vi "joystick and camera_ms.vi"(9 "Tab Control":T2(tab)=enum."motion 2", 10 "Text":string, 11 "controller in":T5={"A3200.lvclass"=refnum, "Ultimus V2.lvclass"=refnum, "NI-DAQ.lvclass"=refnum, "Motion.lvclass"=refnum, "I-O.lvclass"=refnum, "Dispenser.lvclass"=refnum}) -> (2 "Gantry":dbl[](array[numeric]) format="%#_8g", 3 "controller out":T5)   [LabVIEW 2016]
uses:
  Classes/Controller/Motion/A3200 Folder/A3200.lvclass
  D:/Gantry_General/Classes/Controller/Motion/Motion Folder/Motion.lvclass
  Classes/Controller/Dispenser/Ultimus V2 Folder/Ultimus V2.lvclass
  Classes/Controller/I-O/NI-DAQ Folder/NI-DAQ.lvclass
  Classes/Controller/Motion/Motion Folder/Motion.lvclass
  Classes/Controller/I-O/I-O Folder/I-O.lvclass
  Classes/Controller/Dispenser/Dispenser Folder/Dispenser.lvclass
  Classes/Controller/Camera/Camera Folder/Machine Vision.ctl
  Classes/Controller/Camera/Camera Folder/Camera.lvclass
panel:
  out "pass/>(r)/<(-r)":bool[][](array[boolean])
  in  "range(r)":dbl[](array[numeric])=[0.001, 0.001, 0.0, 0.0] format="%#_8g"
  in  "camera on":bool
  in  "Go Gantry position":bool
  out "Gantry poistion":dbl[](array[numeric]) format="%#_8g"
  out "Boolean":bool
  in  "Machine Vision 2":T1=enum."tracker fiducial"
  in  "Machine Vision":T1=enum."None"
  in  "Joystick":bool
  in  "Go sum":bool
  out "Sum":dbl[](array[numeric])=[0.00017791618301998824, 0.0005389674915932119, 0.0, 0.0] format="%#_8g"
  out "Camera":dbl[](array[numeric])=[0.00017791618301998824, 0.0005389674915932119] format="%#_8g"
  in  "Stop":bool
  out "Numeric":dbl
  in  "input":dbl=70.0
  in  "Camera light":bool
  in  "On/Off":bool
  in  "Channel":i32=20
  in  "Vacuum":bool
  in  "Jog Cluster":T3={"Jog XY Cluster"={"object goes up"=FALSE, "object goes down"=FALSE, "object goes right"=FALSE, "object goes left"=FALSE, "SW2"=TRUE, "SW1"=TRUE, "YY (mm)"=0.1, "YN (mm) "=0.01, "NY (mm) "=0.002, "NN (mm) "=0.0005}, "Jog Z Cluster "={"Z go down 0.1 mm"=FALSE, "Z go up 0.1 mm"=FALSE, "Z go down 0.05 mm"=FALSE, "Z go up 0.05 mm"=FALSE, "Z go down 0.01 mm"=FALSE, "Z go up 0.01 mm"=FALSE, "Z go down"=FALSE, "Z go up"=FALSE, "step (mm)"=0.001}}
  in  "XY Speed 2":dbl=20.0
  in  "XY add":dbl[](array[numeric])=[380.0238, 0.0014, 55.58184794305402, -0.0005137759006832702] format="%#_8g"
  in  "get P2 add":bool
  in  "XY go 5":bool
  in  "XY Position 5":dbl[](array[numeric])=[389.0, 389.0, 55.58184800408918, -0.0005138406154977592] format="%#_8g"
  in  "get Postion 5":bool
  in  "XY go 4":bool
  in  "XY Position 4":dbl[](array[numeric])=[592.3687645323295, 397.60426466601484, 55.58184800408918, -0.0005138406154977592] format="%#_8g"
  in  "get Postion 4":bool
  in  "XY go 3":bool
  in  "XY Position 3":dbl[](array[numeric])=[972.3689967686571, 397.60610398471965, 55.58184796594221, -0.0005142432854545792] format="%#_8g"
  in  "get Postion 3":bool
  in  "XY Position 1":dbl[](array[numeric])=[9.0, 9.0, 35.37118150994465, -9.480284627999261e-05] format="%#_8g"
  in  "XY go 1":bool
  in  "Z Position":dbl=35.37
  in  "Z Go":bool
  in  "XY go 2":bool
  in  "XY Position 2":dbl[](array[numeric])=[769.0237955548766, 389.000010557689, 90.95302945299866, -0.0006085787469632629] format="%#_8g"
  in  "get Postion 1":bool
  in  "get Postion 2":bool
  in  "XY Speed":dbl=100.0
  in  "z Speed":dbl=20.0 format="%#_13g"
  in  "add postion":dbl[](array[numeric])=[360.0223, 0.0021, 0.0, 0.0] format="%#_8g"
  in  "get and go Position":T4={"get P Array"=[FALSE, FALSE, FALSE, FALSE, FALSE], "XY go P Array"=[FALSE, FALSE, FALSE, FALSE, FALSE], "xyzu Position Array"=[[369.99999758410644, 730.0222975841064, 0.0, 0.0, 370.0], [370.00000242422084, 370.0021024242208, 0.0, 0.0, 370.0], [35.29999980758057, 35.29999980758057, 0.0, 0.0, 35.3], [-6.534758156392827e-07, -6.534758156392827e-07, 0.0, 0.0, 0.0]], "XYZ go P Array"=[FALSE, FALSE, FALSE, FALSE, FALSE]} {"xyzu Position Array" format="%#_8g"}
  in  "input postion test":dbl[](array[numeric])
  out "Array out":dbl[](array[numeric])=[369.99999758410644, 370.00000242422084]
  out "XY(F)/XYZ(T)":bool
  in  "P2 get P1 add position":bool
  out "Image 2":T6(plugin-control)
  out "Image":T6(plugin-control)
  # "X\nY"
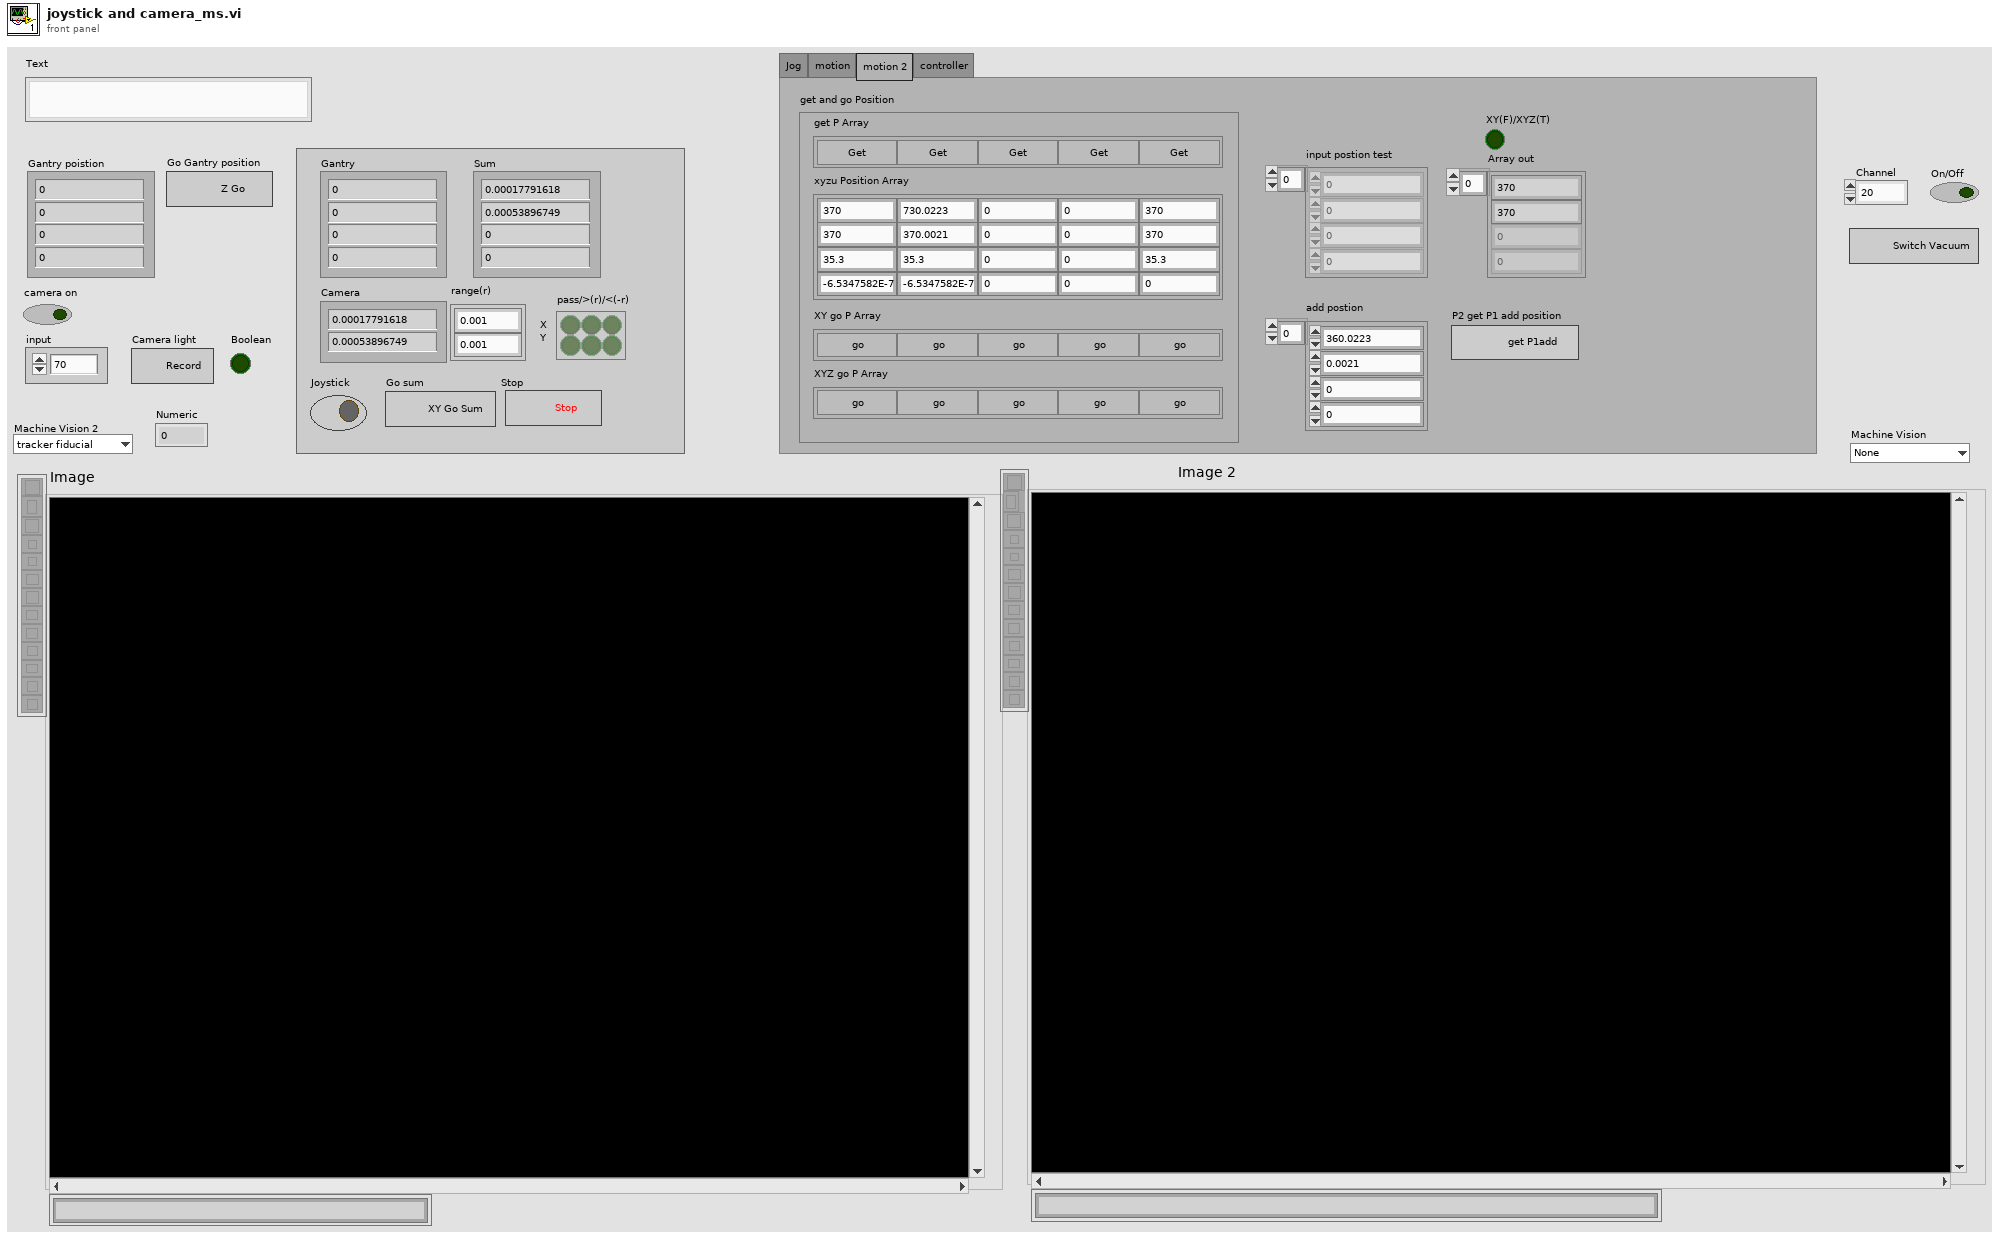
[diagram p1: front panel]
types:
  T1 = typedef "Camera.lvclass/Machine Vision.ctl" = enum16{"top left corner", "top right corner", "bottom left corner", "bottom right corner", "bottom left chip", "top right chip", "None", "tracker fiducial", "chip cross 2", "chip cross", "Focus", "INTT HDI Mark", "INTT Sensor Cross", "INTT Chip Corner", "HPK Silicon", "HPK Silicon square", "8inch PCB Pad ", "8inch PCB Pad2", "Circle", "tpcb_hole"}
  T2 = enum32{"Jog", "motion", "motion 2", "controller"}
  T3 = cluster{"Jog XY Cluster":cluster{"object goes up":bool, "object goes down":bool, "object goes right":bool, "object goes left":bool, "SW2":bool, "SW1":bool, "YY (mm)":dbl, "YN (mm) ":dbl, "NY (mm) ":dbl, "NN (mm) ":dbl}, "Jog Z Cluster ":cluster{"Z go down 0.1 mm":bool, "Z go up 0.1 mm":bool, "Z go down 0.05 mm":bool, "Z go up 0.05 mm":bool, "Z go down 0.01 mm":bool, "Z go up 0.01 mm":bool, "Z go down":bool, "Z go up":bool, "step (mm)":dbl}}
  T4 = cluster{"get P Array":bool[], "XY go P Array":bool[], "xyzu Position Array":dbl[][], "XYZ go P Array":bool[]}
  T5 = cluster{"A3200.lvclass":refnum<class "A3200.lvclass">, "Ultimus V2.lvclass":refnum<class "Ultimus V2.lvclass">, "NI-DAQ.lvclass":refnum<class "NI-DAQ.lvclass">, "Motion.lvclass":refnum<class "Motion.lvclass">, "I-O.lvclass":refnum<class "I-O.lvclass">, "Dispenser.lvclass":refnum<class "Dispenser.lvclass">}
  T6 = typedef "IMAQ Image.ctl" = refnum<image>
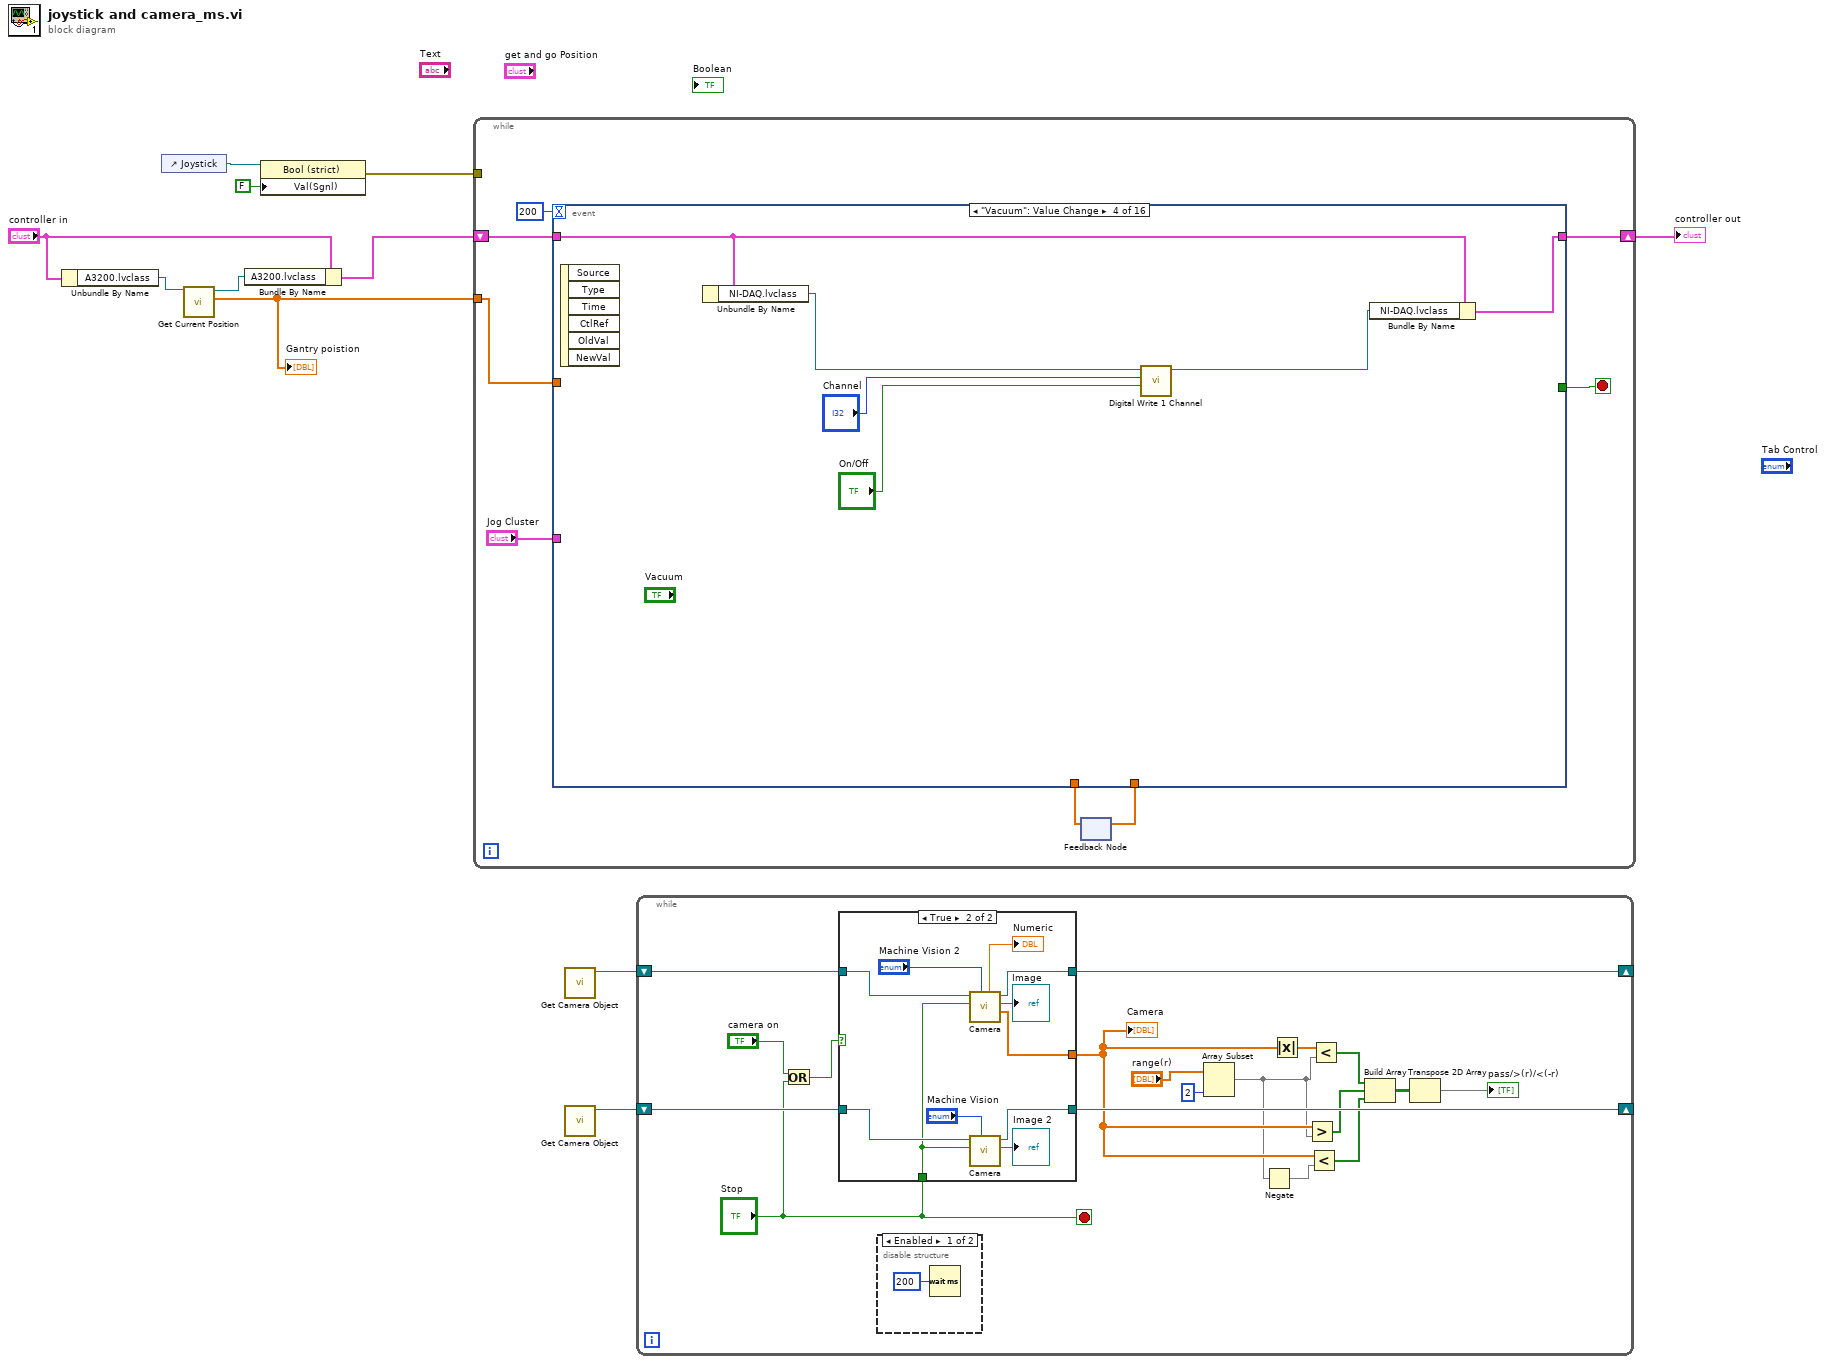
[diagram p0: block diagram]
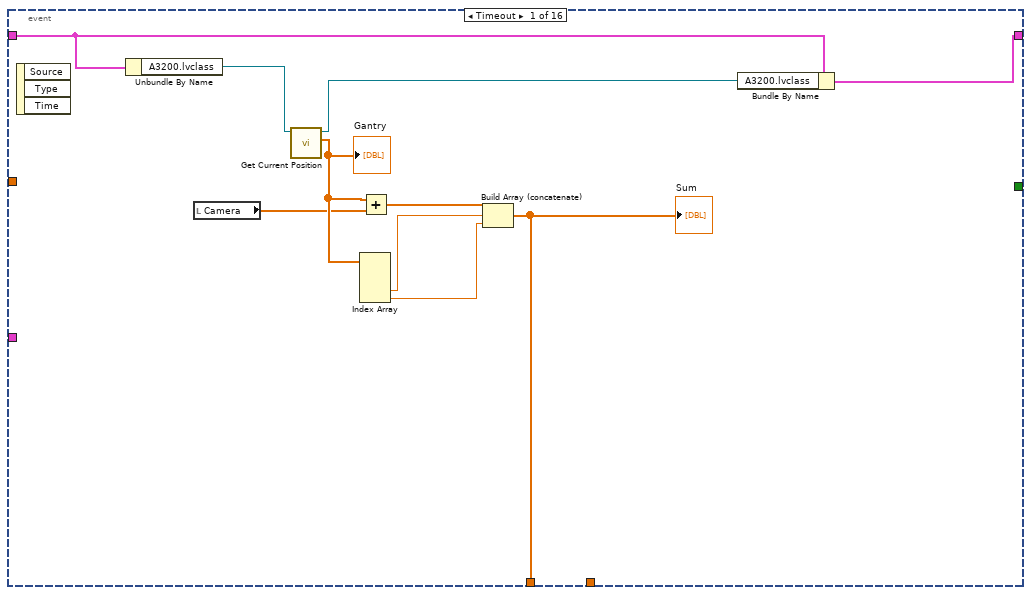
[diagram p2: hidden frame]
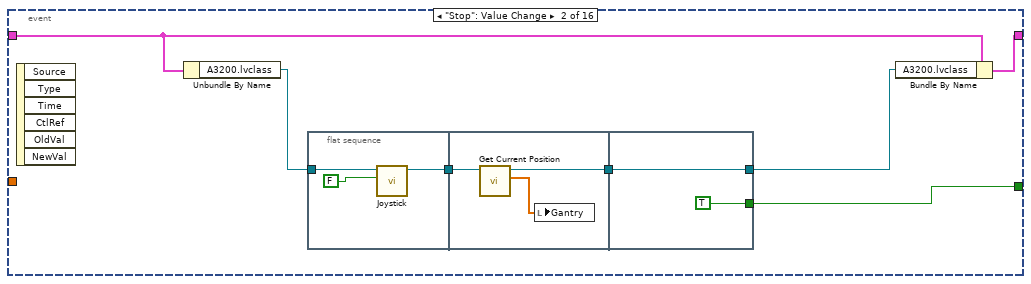
[diagram p3: hidden frame]
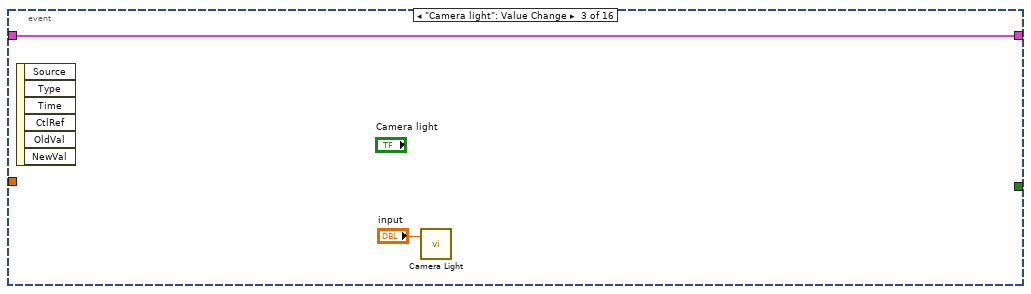
[diagram p4: hidden frame]
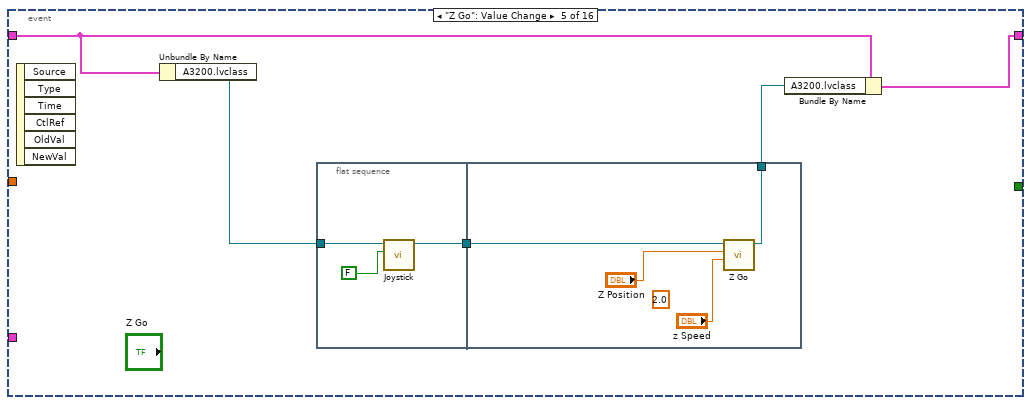
[diagram p5: hidden frame]
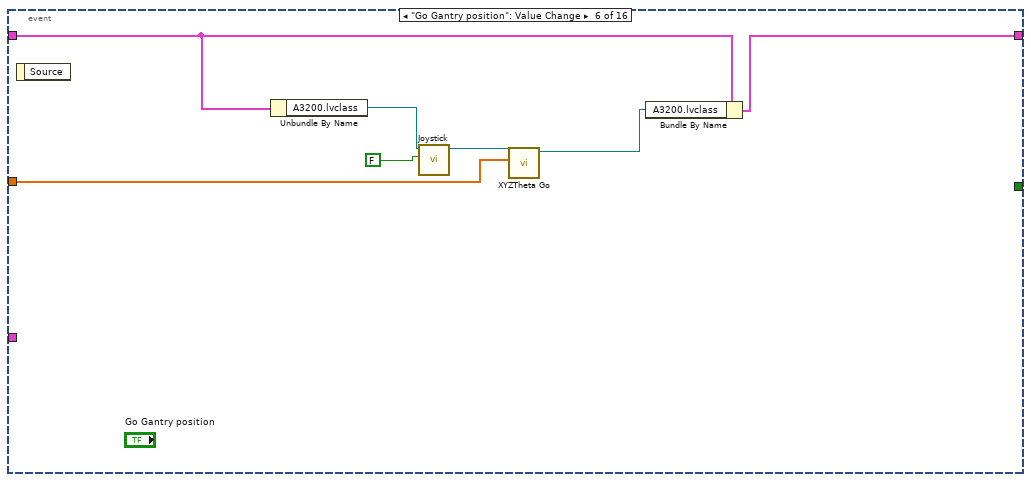
[diagram p6: hidden frame]
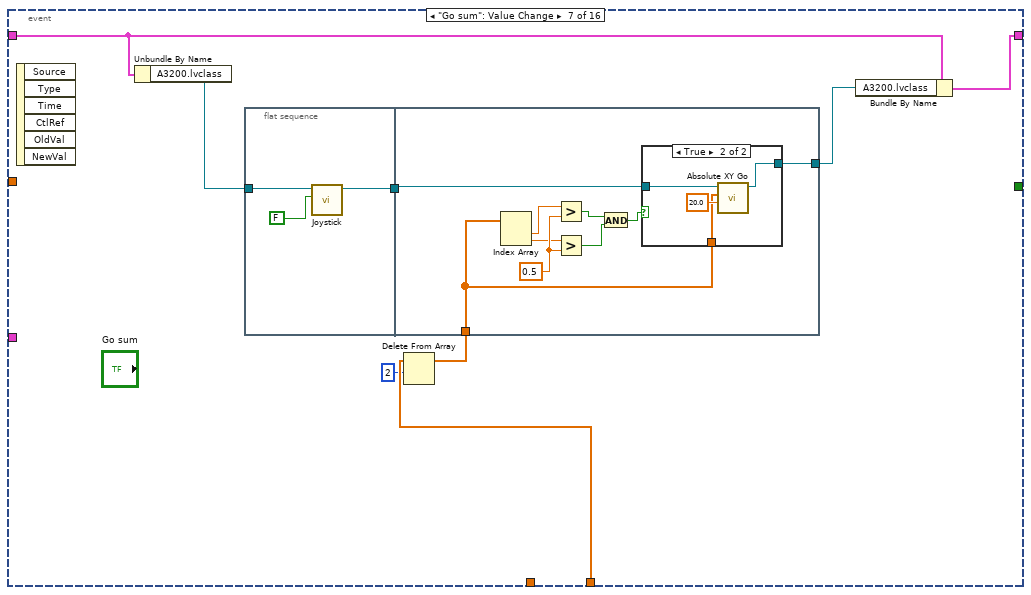
[diagram p7: hidden frame]
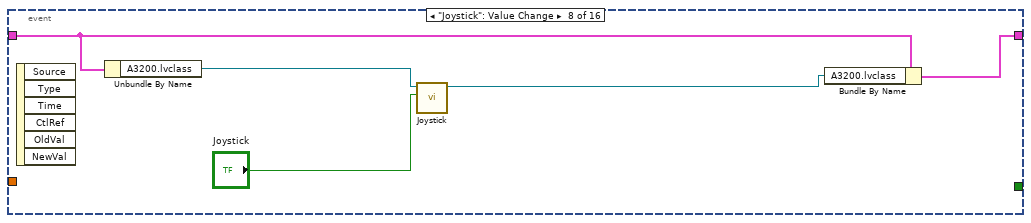
[diagram p9: hidden frame]
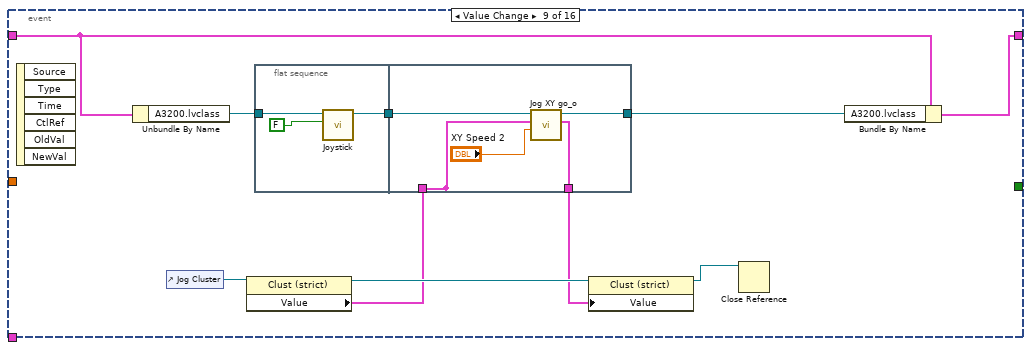
[diagram p10: hidden frame]
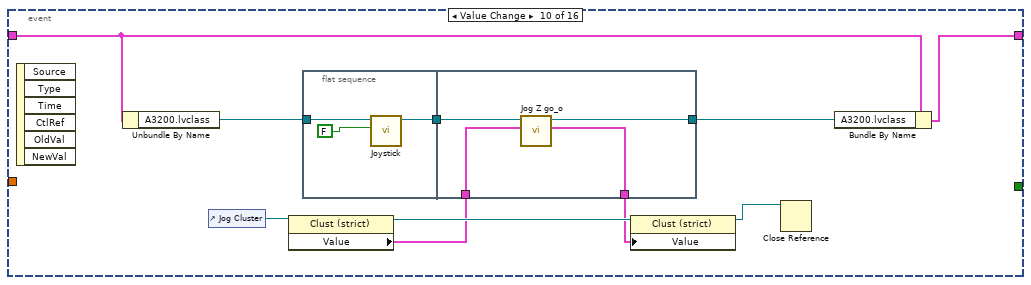
[diagram p11: hidden frame]
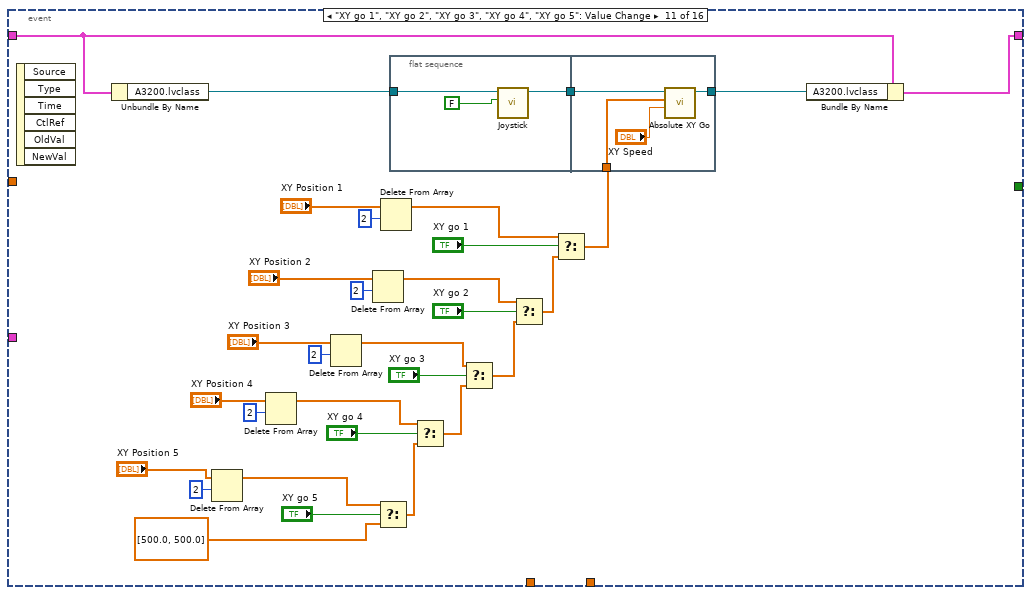
[diagram p12: hidden frame]
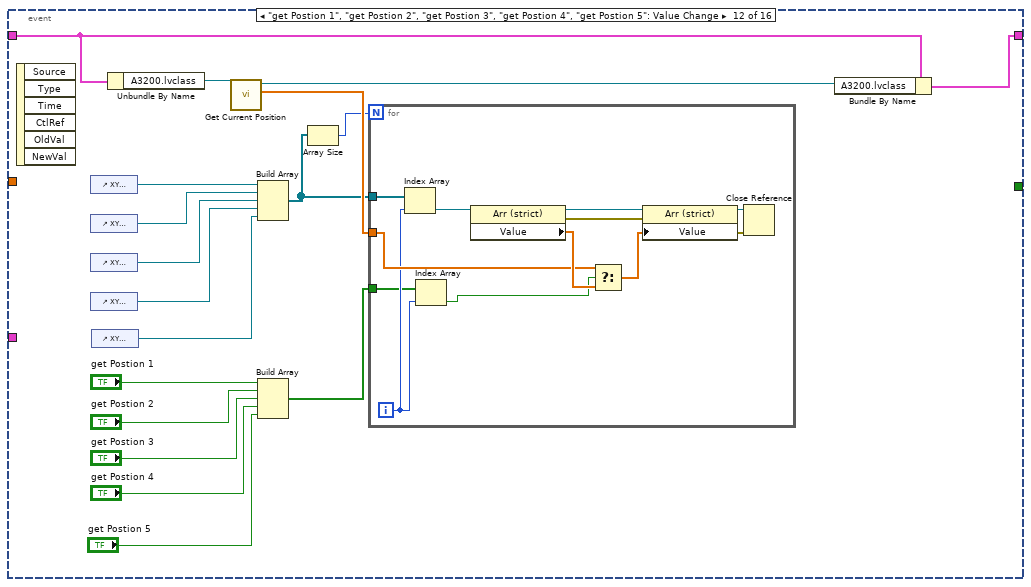
[diagram p13: hidden frame]
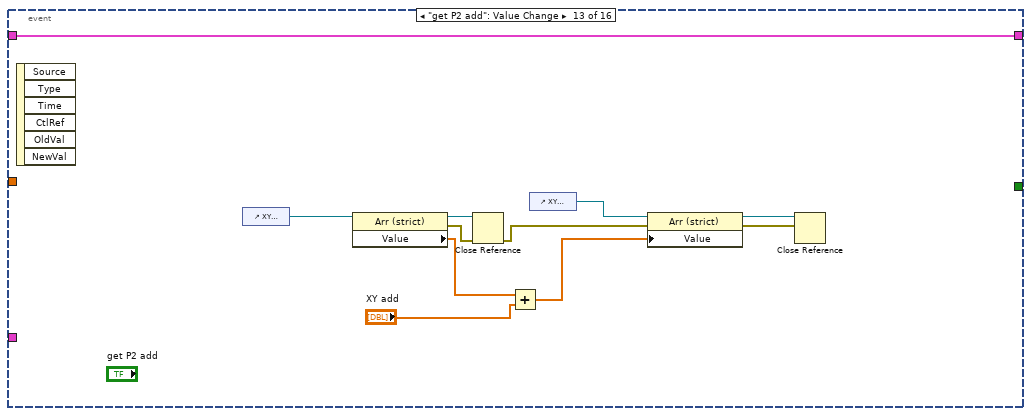
[diagram p14: hidden frame]
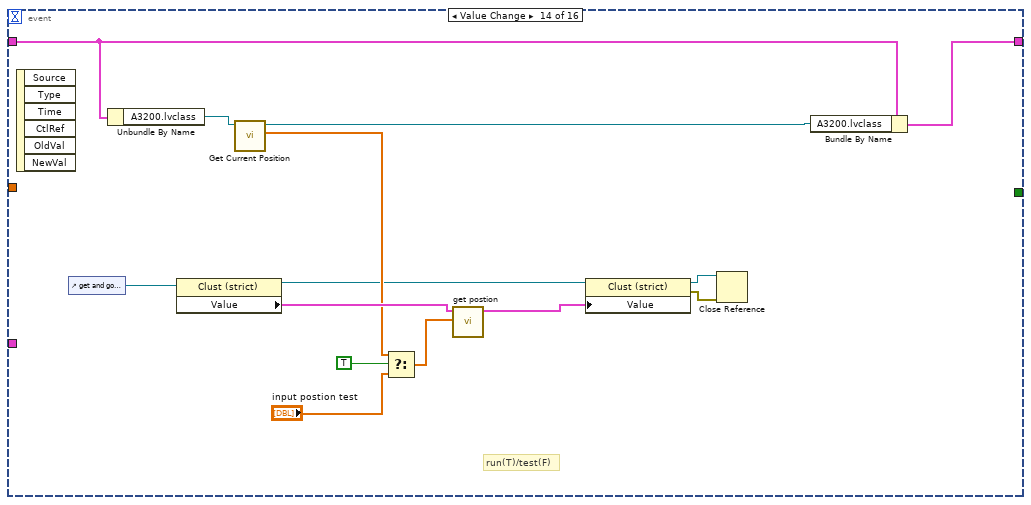
[diagram p15: hidden frame]
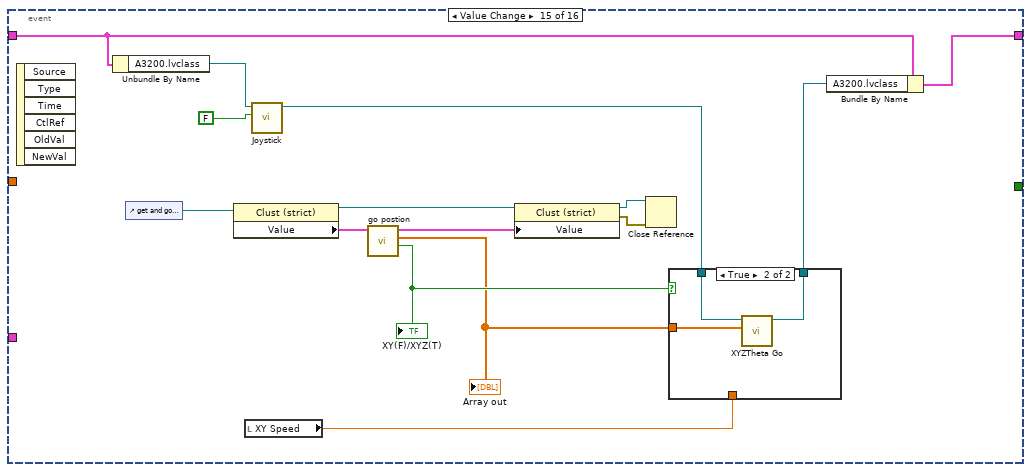
[diagram p16: hidden frame]
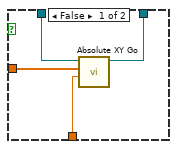
[diagram p17: hidden frame]
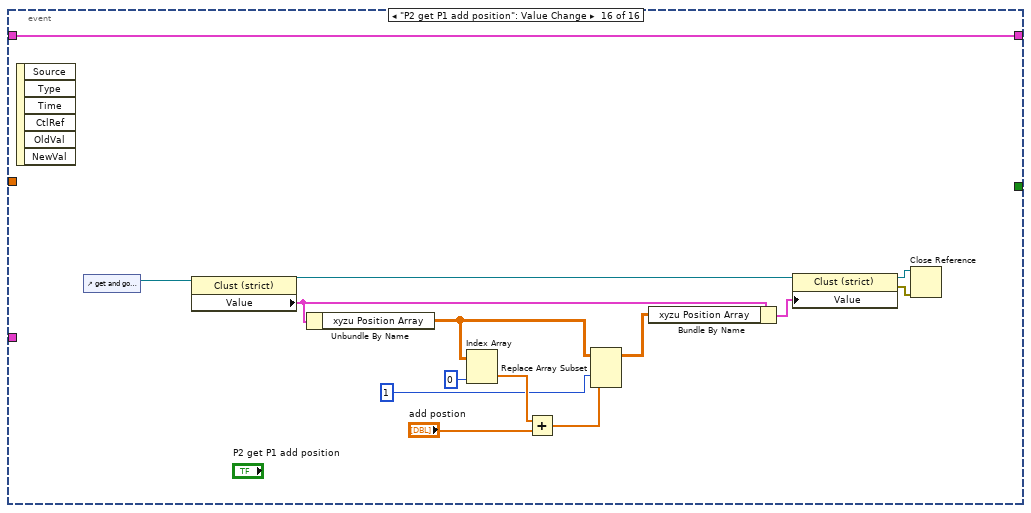
[diagram p18: hidden frame]
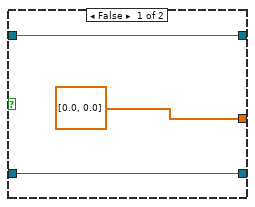
[diagram p19: hidden frame]
diagram:
  n1 = Unbundle By Name("controller in") -> ("A3200.lvclass"=w5:refnum<class "A3200.lvclass">)
  n2 = control-ref of="Joystick"() -> (w8:refnum<vi>)
  n3 = call-dynamic "Get Current Position.vi"("Gantry in"=w5) -> ("XYZTheta Out"=w1:dbl[], "Gantry out"=w4:refnum<class "A3200.lvclass">)  [unwired: 8 in, 1 out]
  "Gantry poistion" <- w1
  n4 = Bundle By Name(cluster="controller in", "A3200.lvclass"=w4) -> (w2:T5)
  n5 = property class="Bool (strict)"(reference=w8, "Val(Sgnl)"=FALSE ("Value (Signaling)")) -> (error out=w7:errorcluster)  [unwired: 1 in, 1 out]
  n6 = while {
    tunnel: w7 -> [_]
    shift-right: [w19] -> w6
    shift-left: w2 -> [w13]
    tunnel: w1 -> [w12]
    stop <- w18 stop-if-true
    n7 = feedback #1() -> (w16:dbl[])  [unwired: 1 in]
    n8 = event shown="[3] \"Vacuum\": Value Change" {
      selector: _ -> [_ _ _ _ _ _ _ _ _ _ _ _ _ _ _ _]
      dyn-events: _ -> [_ _ _ _ _ _ _ _ _ _ _ _ _ _ _ _]
      timeout: 200 -> [_ _ _ _ _ _ _ _ _ _ _ _ _ _ _ _]
      tunnel: [w26 w34 w46 w48 w54 w70 w76 w98 w108 w125 w164 w192 w215 w228 w243 w265] -> w19
      tunnel: w13 -> [w27 w35 w46 w49 w55 w66 w77 w99 w109 w126 w165 w191 w215 w229 w241 w265]
      tunnel: [_ w32 _ _ _ _ _ _ _ _ _ _ _ _ _ _] -> w18
      tunnel: [w22 _ _ _ _ _ _ _ _ _ _ _ _ _ _ _] -> w17
      tunnel: w16 -> [_ _ _ _ _ _ w73 _ _ _ _ _ _ _ _ _]
      tunnel: "Jog Cluster" -> [_ _ _ _ _ _ _ _ _ _ _ _ _ _ _ _]
      tunnel: w12 -> [_ _ _ _ _ w65 _ _ _ _ _ _ _ _ _ _]
      event Timeout {
        n9 = event-data() -> ()  [unwired: 1 in, 3 out]
        n10 = Unbundle By Name(w27) -> ("A3200.lvclass"=w28:refnum<class "A3200.lvclass">)
        n11 = local read "Camera"() -> (w20:dbl[])
        n12 = call-dynamic "Get Current Position.vi"("Gantry in"=w28) -> ("XYZTheta Out"=w25:dbl[], "Gantry out"=w29:refnum<class "A3200.lvclass">)  [unwired: 8 in, 1 out]
        "Gantry" <- w25
        n13 = Index Array(array=w25) -> (element #3=w24:dbl, element #4=w23:dbl)  [unwired: 4 in, 2 out]
        n14 = Add(x=w25, y=w20) -> (x+y=w21:dbl[])
        n15 = Build Array (concatenate)(w21, w24, w23) -> (w22:dbl[])
        "Sum" <- w22
        n16 = Bundle By Name(cluster=w27, "A3200.lvclass"=w29) -> (w26:T5)
      }
      event "Stop": Value Change {
        n17 = event-data() -> ()  [unwired: 1 in, 6 out]
        n18 = Unbundle By Name(w35) -> ("A3200.lvclass"=w36:refnum<class "A3200.lvclass">)
        n19 = flat-sequence {
          tunnel: w36 -> [w38]
          tunnel: [w37] -> w31
          tunnel: w31 -> [w41]
          tunnel: [w40] -> w30
          tunnel: [w44] -> w33
          tunnel: w30 -> [w44]
          tunnel: [TRUE] -> w32
          frame #0 {
            n20 = call-dynamic "Joystick.vi"("Joystick"=FALSE, "Gantry in"=w38) -> ("Gantry out"=w37:refnum<class "A3200.lvclass">)  [unwired: 8 in, 1 out]
          }
          frame #1 {
            n21 = call-dynamic "Get Current Position.vi"("Gantry in"=w41) -> ("XYZTheta Out"=w42:dbl[], "Gantry out"=w40:refnum<class "A3200.lvclass">)  [unwired: 8 in, 1 out]
            n22 = local write "Gantry"(w42) -> ()
          }
          frame #2 {
          }
        }
        n23 = Bundle By Name(cluster=w35, "A3200.lvclass"=w33) -> (w34:T5)
      }
      event "Camera light": Value Change {
        n24 = event-data() -> ()  [unwired: 1 in, 6 out]
        n25 = call "Camera Light.vi"("input"="input") -> ()  [unwired: 2 in, 1 out]
      }
      event "Vacuum": Value Change {
        n26 = event-data() -> ()  [unwired: 1 in, 6 out]
        n27 = Unbundle By Name(w49) -> ("NI-DAQ.lvclass"=w50:refnum<class "NI-DAQ.lvclass">)
        n28 = call-dynamic "Digital Write 1 Channel.vi"("Value"="On/Off", "Channel"="Channel", "NI-DAQ.lvclass"=w50) -> ("NI-DAQ.lvclass 2"=w47:refnum<class "NI-DAQ.lvclass">)  [unwired: 7 in, 1 out]
        n29 = Bundle By Name(cluster=w49, "NI-DAQ.lvclass"=w47) -> (w48:T5)
      }
      event "Z Go": Value Change {
        n30 = event-data() -> ()  [unwired: 1 in, 6 out]
        n31 = Unbundle By Name(w55) -> ("A3200.lvclass"=w56:refnum<class "A3200.lvclass">)
        n32 = flat-sequence {
          tunnel: w56 -> [w58]
          tunnel: [w59] -> w53
          tunnel: [w63] -> w57
          tunnel: w53 -> [w62]
          frame #0 {
            n33 = call-dynamic "Joystick.vi"("Joystick"=FALSE, "Gantry in"=w58) -> ("Gantry out"=w59:refnum<class "A3200.lvclass">)  [unwired: 8 in, 1 out]
          }
          frame #1 {
            (unwired) 2.0 ("Speed")
            n34 = call-dynamic "Z Go.vi"("Speed"="z Speed", "Position"="Z Position", "Gantry in"=w62) -> ("Gantry out"=w63:refnum<class "A3200.lvclass">)  [unwired: 7 in, 1 out]
          }
        }
        n35 = Bundle By Name(cluster=w55, "A3200.lvclass"=w57) -> (w54:T5)
      }
      event "Go Gantry position": Value Change {
        n36 = event-data() -> ()  [unwired: 1 in, 1 out]
        n37 = Unbundle By Name(w66) -> ("A3200.lvclass"=w68:refnum<class "A3200.lvclass">)
        n38 = call-dynamic "Joystick.vi"("Joystick"=FALSE, "Gantry in"=w68) -> ("Gantry out"=w67:refnum<class "A3200.lvclass">)  [unwired: 8 in, 1 out]
        n39 = call "XYZTheta Go.vi"("XYZTheta In"=w65, "Motion in"=w67) -> ("Motion out"=w69:refnum<class "A3200.lvclass">)  [unwired: 7 in, 2 out]
        n40 = Bundle By Name(cluster=w66, "A3200.lvclass"=w69) -> (w70:T5)
      }
      event "Go sum": Value Change {
        n41 = event-data() -> ()  [unwired: 1 in, 6 out]
        n42 = Unbundle By Name(w77) -> ("A3200.lvclass"=w78:refnum<class "A3200.lvclass">)
        n43 = flat-sequence {
          tunnel: w78 -> [w80]
          tunnel: [w81] -> w79
          tunnel: w79 -> [w91]
          tunnel: [w90] -> w75
          tunnel: w74 -> [w83]
          frame #0 {
            n44 = call-dynamic "Joystick.vi"("Joystick"=FALSE, "Gantry in"=w80) -> ("Gantry out"=w81:refnum<class "A3200.lvclass">)  [unwired: 8 in, 1 out]
          }
          frame #1 {
            w86 = 0.5 ("y")
            n45 = Index Array(array=w83) -> (element #1=w84:dbl, element #2=w85:dbl)  [unwired: 2 in]
            n46 = Greater?(x=w84, y=w86) -> (0:w88:bool)
            n47 = Greater?(x=w85, y=w86) -> (0:w87:bool)
            n48 = And(x=w88, y=w87) -> (x .and. y?=w89:bool)
            n49 = case shown="True" w89 {
              tunnel: w91 -> [w92 w96]
              tunnel: [w92 w95] -> w90
              tunnel: w83 -> [_ w93]
              frame False {
              }
              frame True {
                n50 = call-dynamic "Absolute XY Go.vi"("Speed"=20.0, "XY"=w93, "Gantry in"=w96) -> ("Gantry out"=w95:refnum<class "A3200.lvclass">)  [unwired: 7 in, 1 out]
              }
            }
          }
        }
        n51 = Delete From Array(array=w73, length=2) -> (array with subset deleted=w74:dbl[])  [unwired: 1 in, 1 out]
        n52 = Bundle By Name(cluster=w77, "A3200.lvclass"=w75) -> (w76:T5)
      }
      event "Joystick": Value Change {
        n53 = event-data() -> ()  [unwired: 1 in, 6 out]
        n54 = Unbundle By Name(w99) -> ("A3200.lvclass"=w97:refnum<class "A3200.lvclass">)
        n55 = call-dynamic "Joystick.vi"("Joystick"="Joystick", "Gantry in"=w97) -> ("Gantry out"=w101:refnum<class "A3200.lvclass">)  [unwired: 8 in, 1 out]
        n56 = Bundle By Name(cluster=w99, "A3200.lvclass"=w101) -> (w98:T5)
      }
      event "Jog Cluster.Jog XY Cluster.object goes up", "Jog Cluster.Jog XY Cluster.object goes down", "Jog Cluster.Jog XY Cluster.object goes right", "Jog Cluster.Jog XY Cluster.object goes left": Value Change {
        n57 = event-data() -> ()  [unwired: 1 in, 6 out]
        n58 = Unbundle By Name(w109) -> ("A3200.lvclass"=w111:refnum<class "A3200.lvclass">)
        n59 = control-ref of="Jog Cluster"() -> (w104:refnum<vi>)
        n60 = property class="Clust (strict)"(reference=w104) -> (reference out=w105:refnum<vi>, "Value"=w103:T3)  [unwired: 1 in, 1 out]
        n61 = flat-sequence {
          tunnel: w111 -> [w113]
          tunnel: [w112] -> w107
          tunnel: w107 -> [w119]
          tunnel: [w117] -> _
          tunnel: [w118] -> w110
          tunnel: w103 -> [w117]
          tunnel: [w115] -> w102
          frame #0 {
            n62 = call-dynamic "Joystick.vi"("Joystick"=FALSE, "Gantry in"=w113) -> ("Gantry out"=w112:refnum<class "A3200.lvclass">)  [unwired: 8 in, 1 out]
          }
          frame #1 {
            n63 = call "Jog XY go_o.vi"("Speed"="XY Speed 2", "Jog Cluster"=w117, "A3200.lvclass IN"=w119) -> ("Jog Cluster output"=w115:T3, "A3200.lvclass OUT"=w118:refnum<class "A3200.lvclass">)  [unwired: 7 in]
          }
        }
        n64 = property class="Clust (strict)"(reference=w105, "Value"=w102) -> (reference out=w106:refnum<vi>)  [unwired: 1 in, 1 out]
        n65 = Close Reference(reference=w106) -> ()  [unwired: 1 in, 1 out]
        n66 = Bundle By Name(cluster=w109, "A3200.lvclass"=w110) -> (w108:T5)
      }
      event "Jog Cluster.Jog Z Cluster.Z go down 0.1 mm", "Jog Cluster.Jog Z Cluster.Z go up 0.1 mm", "Jog Cluster.Jog Z Cluster.Z go down 0.05 mm", "Jog Cluster.Jog Z Cluster.Z go up 0.05 mm", "Jog Cluster.Jog Z Cluster.Z go down 0.01 mm", "Jog Cluster.Jog Z Cluster.Z go up 0.01 mm", "Jog Cluster.Jog Z Cluster.Z go down", "Jog Cluster.Jog Z Cluster.Z go up": Value Change {
        n67 = event-data() -> ()  [unwired: 1 in, 6 out]
        n68 = Unbundle By Name(w126) -> ("A3200.lvclass"=w128:refnum<class "A3200.lvclass">)
        n69 = control-ref of="Jog Cluster"() -> (w122:refnum<vi>)
        n70 = property class="Clust (strict)"(reference=w122) -> (reference out=w123:refnum<vi>, "Value"=w121:T3)  [unwired: 1 in, 1 out]
        n71 = flat-sequence {
          tunnel: w128 -> [w131]
          tunnel: [w130] -> w129
          tunnel: w129 -> [w136]
          tunnel: w121 -> [w134]
          tunnel: [w135] -> w127
          tunnel: [w133] -> w120
          frame #0 {
            n72 = call-dynamic "Joystick.vi"("Joystick"=FALSE, "Gantry in"=w131) -> ("Gantry out"=w130:refnum<class "A3200.lvclass">)  [unwired: 8 in, 1 out]
          }
          frame #1 {
            n73 = call "Jog Z go_o.vi"("Jog Cluster"=w134, "A3200.lvclass IN"=w136) -> ("Jog Cluster output"=w133:T3, "A3200.lvclass OUT"=w135:refnum<class "A3200.lvclass">)  [unwired: 8 in]
          }
        }
        n74 = property class="Clust (strict)"(reference=w123, "Value"=w120) -> (reference out=w124:refnum<vi>)  [unwired: 1 in, 1 out]
        n75 = Close Reference(reference=w124) -> ()  [unwired: 1 in, 1 out]
        n76 = Bundle By Name(cluster=w126, "A3200.lvclass"=w127) -> (w125:T5)
      }
      event "XY go 1", "XY go 2", "XY go 3", "XY go 4", "XY go 5": Value Change {
        n77 = event-data() -> ()  [unwired: 1 in, 6 out]
        n78 = Unbundle By Name(w165) -> ("A3200.lvclass"=w167:refnum<class "A3200.lvclass">)
        n79 = Delete From Array(array="XY Position 5", length=2) -> (array with subset deleted=w137:dbl[])  [unwired: 1 in, 1 out]
        n80 = Delete From Array(array="XY Position 4", length=2) -> (array with subset deleted=w149:dbl[])  [unwired: 1 in, 1 out]
        n81 = Delete From Array(array="XY Position 3", length=2) -> (array with subset deleted=w152:dbl[])  [unwired: 1 in, 1 out]
        n82 = Delete From Array(array="XY Position 2", length=2) -> (array with subset deleted=w153:dbl[])  [unwired: 1 in, 1 out]
        n83 = Select(t=w137, s="XY go 5", f=dbl[] [500.0, 500.0]) -> (s? t:f=w142:dbl[])
        n84 = Delete From Array(array="XY Position 1", length=2) -> (array with subset deleted=w158:dbl[])  [unwired: 1 in, 1 out]
        n85 = flat-sequence {
          tunnel: w167 -> [w169]
          tunnel: [w168] -> w160
          tunnel: [w173] -> w166
          tunnel: w160 -> [w174]
          tunnel: w159 -> [w172]
          frame #0 {
            n86 = call-dynamic "Joystick.vi"("Joystick"=FALSE, "Gantry in"=w169) -> ("Gantry out"=w168:refnum<class "A3200.lvclass">)  [unwired: 8 in, 1 out]
          }
          frame #1 {
            n87 = call-dynamic "Absolute XY Go.vi"("Speed"="XY Speed", "XY"=w172, "Gantry in"=w174) -> ("Gantry out"=w173:refnum<class "A3200.lvclass">)  [unwired: 7 in, 1 out]
          }
        }
        n88 = Select(t=w149, s="XY go 4", f=w142) -> (s? t:f=w148:dbl[])
        n89 = Select(t=w152, s="XY go 3", f=w148) -> (s? t:f=w147:dbl[])
        n90 = Select(t=w153, s="XY go 2", f=w147) -> (s? t:f=w163:dbl[])
        n91 = Select(t=w158, s="XY go 1", f=w163) -> (s? t:f=w159:dbl[])
        n92 = Bundle By Name(cluster=w165, "A3200.lvclass"=w166) -> (w164:T5)
      }
      event "get Postion 1", "get Postion 2", "get Postion 3", "get Postion 4", "get Postion 5": Value Change {
        n93 = event-data() -> ()  [unwired: 1 in, 6 out]
        n94 = control-ref of="XY Position 1"() -> (w184:refnum<vi>)
        n95 = control-ref of="XY Position 2"() -> (w187:refnum<vi>)
        n96 = control-ref of="XY Position 3"() -> (w186:refnum<vi>)
        n97 = control-ref of="XY Position 4"() -> (w185:refnum<vi>)
        n98 = control-ref of="XY Position 5"() -> (w175:refnum<vi>)
        n99 = Unbundle By Name(w191) -> ("A3200.lvclass"=w190:refnum<class "A3200.lvclass">)
        n100 = call-dynamic "Get Current Position.vi"("Gantry in"=w190) -> ("XYZTheta Out"=w188:dbl[], "Gantry out"=w189:refnum<class "A3200.lvclass">)  [unwired: 8 in, 1 out]
        n101 = Build Array(w184, w187, w186, w185, w175) -> (w182:refnum<vi>[])
        n102 = Build Array("get Postion 1", "get Postion 2", "get Postion 3", "get Postion 4", "get Postion 5") -> (w181:bool[])
        n103 = Array Size(array=w182) -> (size(s)=w183:i32)
        n104 = for {
          N: w183 -> [_]
          tunnel: w188 -> [w198]
          tunnel: w182 -> [w197]
          tunnel: w181 -> [w193]
          i -> [w194]
          n105 = Index Array(array=w197, index=w194) -> (element=w196:refnum<vi>)
          n106 = Index Array(array=w193, index=w194) -> (element=w195:bool)
          n107 = property class="Arr (strict)"(reference=w196) -> (reference out=w203:refnum<vi>, error out=w204:errorcluster, "Value"=w199:dbl[])  [unwired: 1 in]
          n108 = Select(t=w198, s=w195, f=w199) -> (s? t:f=w200:dbl[])
          n109 = property class="Arr (strict)"(reference=w203, error in=w204, "Value"=w200) -> (reference out=w202:refnum<vi>, error out=w201:errorcluster)
          n110 = Close Reference(reference=w202, error in (no error)=w201) -> ()  [unwired: 1 out]
        }
        n111 = Bundle By Name(cluster=w191, "A3200.lvclass"=w189) -> (w192:T5)
      }
      event "get P2 add": Value Change {
        n112 = event-data() -> ()  [unwired: 1 in, 6 out]
        n113 = control-ref of="XY Position 1"() -> (w208:refnum<vi>)
        n114 = property class="Arr (strict)"(reference=w208) -> (reference out=w207:refnum<vi>, error out=w206:errorcluster, "Value"=w211:dbl[])  [unwired: 1 in]
        n115 = Close Reference(reference=w207, error in (no error)=w206) -> (error out=w205:errorcluster)
        n116 = Add(x=w211, y="XY add") -> (x+y=w210:dbl[])
        n117 = control-ref of="XY Position 2"() -> (w209:refnum<vi>)
        n118 = property class="Arr (strict)"(reference=w209, error in=w205, "Value"=w210) -> (reference out=w214:refnum<vi>, error out=w213:errorcluster)
        n119 = Close Reference(reference=w214, error in (no error)=w213) -> ()  [unwired: 1 out]
      }
      event "get and go Position.get P Array": Value Change {
        # "run(T)/test(F)"
        n120 = event-data() -> ()  [unwired: 1 in, 6 out]
        n121 = control-ref of="get and go Position"() -> (w225:refnum<vi>)
        n122 = Unbundle By Name(w229) -> ("A3200.lvclass"=w227:refnum<class "A3200.lvclass">)
        n123 = property class="Clust (strict)"(reference=w225) -> (reference out=w218:refnum<vi>, "Value"=w223:T4)  [unwired: 1 in, 1 out]
        n124 = call-dynamic "Get Current Position.vi"("Gantry in"=w227) -> ("XYZTheta Out"=w219:dbl[], "Gantry out"=w226:refnum<class "A3200.lvclass">)  [unwired: 8 in, 1 out]
        n125 = Select(t=w219, s=TRUE, f="input postion test") -> (s? t:f=w220:dbl[])
        n126 = call "get postion.vi"("Array"=w220, "get and go Position in"=w223) -> ("get and go Position out"=w224:T4)  [unwired: 9 in]
        n127 = property class="Clust (strict)"(reference=w218, "Value"=w224) -> (reference out=w216:refnum<vi>, error out=w217:errorcluster)  [unwired: 1 in]
        n128 = Close Reference(reference=w216, error in (no error)=w217) -> ()  [unwired: 1 out]
        n129 = Bundle By Name(cluster=w229, "A3200.lvclass"=w226) -> (w228:T5)
      }
      event "get and go Position.XY go P Array", "get and go Position.XYZ go P Array": Value Change {
        n130 = event-data() -> ()  [unwired: 1 in, 6 out]
        n131 = Unbundle By Name(w241) -> ("A3200.lvclass"=w242:refnum<class "A3200.lvclass">)
        n132 = control-ref of="get and go Position"() -> (w240:refnum<vi>)
        n133 = property class="Clust (strict)"(reference=w240) -> (reference out=w237:refnum<vi>, "Value"=w236:T4)  [unwired: 1 in, 1 out]
        n134 = local read "XY Speed"() -> (w230:dbl)
        n135 = call-dynamic "Joystick.vi"("Joystick"=FALSE, "Gantry in"=w242) -> ("Gantry out"=w233:refnum<class "A3200.lvclass">)  [unwired: 8 in, 1 out]
        n136 = call "go postion.vi"("get and go Position in"=w236) -> ("XY(F)/XYZ(T)"=w234:bool, "Array out"=w231:dbl[], "get and go Position out"=w235:T4)  [unwired: 8 in]
        "XY(F)/XYZ(T)" <- w234
        "Array out" <- w231
        n137 = property class="Clust (strict)"(reference=w237, "Value"=w235) -> (reference out=w238:refnum<vi>, error out=w239:errorcluster)  [unwired: 1 in]
        n138 = Close Reference(reference=w238, error in (no error)=w239) -> ()  [unwired: 1 out]
        n139 = case shown="True" w234 {
          tunnel: w233 -> [w246 w251]
          tunnel: [w245 w250] -> w232
          tunnel: w231 -> [w248 w249]
          tunnel: w230 -> [w247 _]
          frame False {
            n140 = call-dynamic "Absolute XY Go.vi"("Speed"=w247, "XY"=w248, "Gantry in"=w246) -> ("Gantry out"=w245:refnum<class "A3200.lvclass">)  [unwired: 7 in, 1 out]
          }
          frame True {
            n141 = call "XYZTheta Go.vi"("XYZTheta In"=w249, "Motion in"=w251) -> ("Motion out"=w250:refnum<class "A3200.lvclass">)  [unwired: 7 in, 2 out]
          }
        }
        n142 = Bundle By Name(cluster=w241, "A3200.lvclass"=w232) -> (w243:T5)
      }
      event "P2 get P1 add position": Value Change {
        n143 = event-data() -> ()  [unwired: 1 in, 6 out]
        n144 = control-ref of="get and go Position"() -> (w264:refnum<vi>)
        n145 = property class="Clust (strict)"(reference=w264) -> (reference out=w254:refnum<vi>, "Value"=w258:T4)  [unwired: 1 in, 1 out]
        n146 = Unbundle By Name(w258) -> ("xyzu Position Array"=w261:dbl[][])
        n147 = Index Array "Index Array"(array=w261, index (col)=0 ("disabled index (col)")) -> (element=w263:dbl[])  [unwired: 1 in]
        n148 = Add(x=w263, y="add postion") -> (x+y=w259:dbl[])
        n149 = Replace Array Subset(array=w261, new element=w259, index (col)=1 ("disabled index (col)")) -> (w257:dbl[][])  [unwired: 1 in]
        n150 = Bundle By Name(cluster=w258, "xyzu Position Array"=w257) -> (w253:T4)
        n151 = property class="Clust (strict)"(reference=w254, "Value"=w253) -> (reference out=w255:refnum<vi>, error out=w256:errorcluster)  [unwired: 1 in]
        n152 = Close Reference(reference=w255, error in (no error)=w256) -> ()  [unwired: 1 out]
      }
    }
    n153 = feedback-in #1(w17) -> ()
  }
  "controller out" <- w6
  n154 = call "Get Camera Object.vi"() -> ("Camera out"=w11:refnum<class "Camera.lvclass">)  [unwired: 10 in, 1 out]
  n155 = call "Get Camera Object.vi"() -> ("Camera out"=w10:refnum<class "Camera.lvclass">)  [unwired: 10 in, 1 out]
  n156 = while {
    shift-right: [w282] -> _
    shift-left: w11 -> [w283]
    shift-right: [w281] -> _
    shift-left: w10 -> [w280]
    stop <- "Stop" stop-if-true
    n157 = Or(x="camera on", y="Stop") -> (x .or. y?=w277:bool)
    n158 = case shown="True" w277 {
      tunnel: w283 -> [w286 w297]
      tunnel: [w286 w296] -> w282
      tunnel: [w285 w294] -> w281
      tunnel: w280 -> [w285 w291]
      tunnel: "Stop" -> [_ w290]
      tunnel: [dbl[] [0.0, 0.0] ("Camera") w287] -> w270
      frame False {
      }
      frame True {
        n159 = call "Camera.vi"("Machine Vision"="Machine Vision 2", "Stop"=w290, "Camera in"=w297) -> ("Camera"=w287:dbl[], "Image"=→"Image":T6, "Camera out"=w296:refnum<class "Camera.lvclass">, "Focus output"=→"Numeric":dbl)  [unwired: 4 in, 1 out]
        n160 = call "Camera.vi"("Machine Vision"="Machine Vision", "Stop"=w290, "Camera in"=w291) -> ("Image"=→"Image 2":T6, "Camera out"=w294:refnum<class "Camera.lvclass">)  [unwired: 4 in, 3 out]
      }
    }
    "Camera" <- w270
    n161 = disable-structure shown="Enabled" {
      frame Enabled {
        n162 = Wait (ms)(milliseconds to wait=u32 200) -> ()  [unwired: 1 out]
      }
      frame Disabled {
      }
    }
    n163 = Array Subset(array="range(r)", length=2) -> (w268:dbl[])  [unwired: 1 in]
    n164 = Negate(x=w268) -> (-x=w269:dbl[])
    n165 = Absolute Value(x=w270) -> (abs(x)=w276:dbl[])
    n166 = Greater?(x=w270, y=w268) -> (0:w266:bool[])
    n167 = Less?(x=w270, y=w269) -> (x < y?=w267:bool[])
    n168 = Less?(x=w276, y=w268) -> (x < y?=w273:bool[])
    n169 = Build Array(w273, w266, w267) -> (w272:bool[][])
    n170 = Transpose 2D Array(2D array=w272) -> (transposed array=→"pass/>(r)/<(-r)":bool[][])
  }
